vi "Format SQL Date.vi"(9 "Month":i16, 11 "YYYY":i32) -> (3 "YYYY-MM-%":string)   [LabVIEW 2018, in "Budgetizer.lvclass"]
uses:
  Budgetizer.lvclass
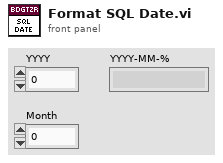
[diagram p1: front panel]
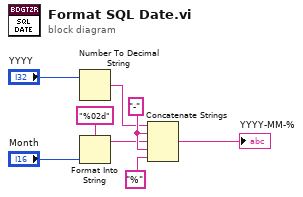
[diagram p0: block diagram]
diagram:
  w4 = "-" ("string")
  n1 = Number To Decimal String(number="YYYY") -> (decimal integer string=w1:string)  [unwired: 1 in]
  n2 = Format Into String(format string="%02d" ("string"), "Month") -> (resulting string=w3:string)  [unwired: 2 in, 1 out]
  n3 = Concatenate Strings(w1, w4, w3, w4, "%" ("string")) -> (→"YYYY-MM-%":string)
